vi "check internet access (tcp).vi"(8 "error in (no error)":errorcluster) -> (0 "error out":errorcluster, 3 "Internet OK":bool)   [LabVIEW 2022 SP3]
panel:
  # "check Internet access (tcp)"
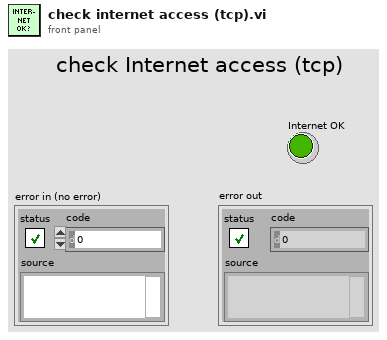
[diagram p1: front panel]
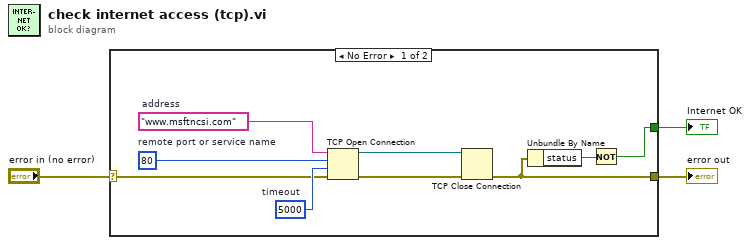
[diagram p0: block diagram]
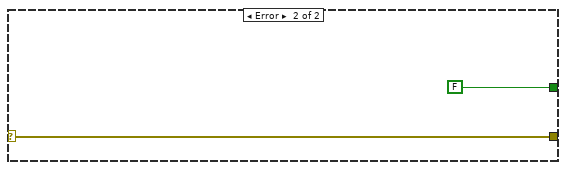
[diagram p2: hidden frame]
diagram:
  n1 = case shown="No Error" "error in (no error)" {
    selector: "error in (no error)" -> [w9 w13]
    tunnel: [w4 FALSE] -> w3
    tunnel: [w6 w13] -> w2
    frame No Error {
      w12 = u16 80  # remote port or service name
      w11 = "www.msftncsi.com"  # address
      w10 = 5000  # timeout
      n2 = TCP Open Connection(address=w11, remote port or service name=w12, timeout ms (60000)=w10, error in (no error)=w9) -> (connection ID=w7:refnum<k5>, error out=w8:errorcluster)  [unwired: 1 in]
      n3 = TCP Close Connection(connection ID=w7, error in (no error)=w8) -> (error out=w6:errorcluster)  [unwired: 1 in, 1 out]
      n4 = Unbundle By Name(w6) -> ("status"=w5:bool)
      n5 = Not(x=w5) -> (.not. x?=w4:bool)
    }
    frame Error {
    }
  }
  "Internet OK" <- w3
  "error out" <- w2
